vi "MeasConfigType_to_Byte.vi"(4 "MeasConfigType":T1) -> (1 "Byte Array":u8[](array[numeric]))   [LabVIEW 2020, in "Avantes.lvclass"]
uses:
  <instrlib>/Classes/CCD/Avantes/Avantes.lvclass
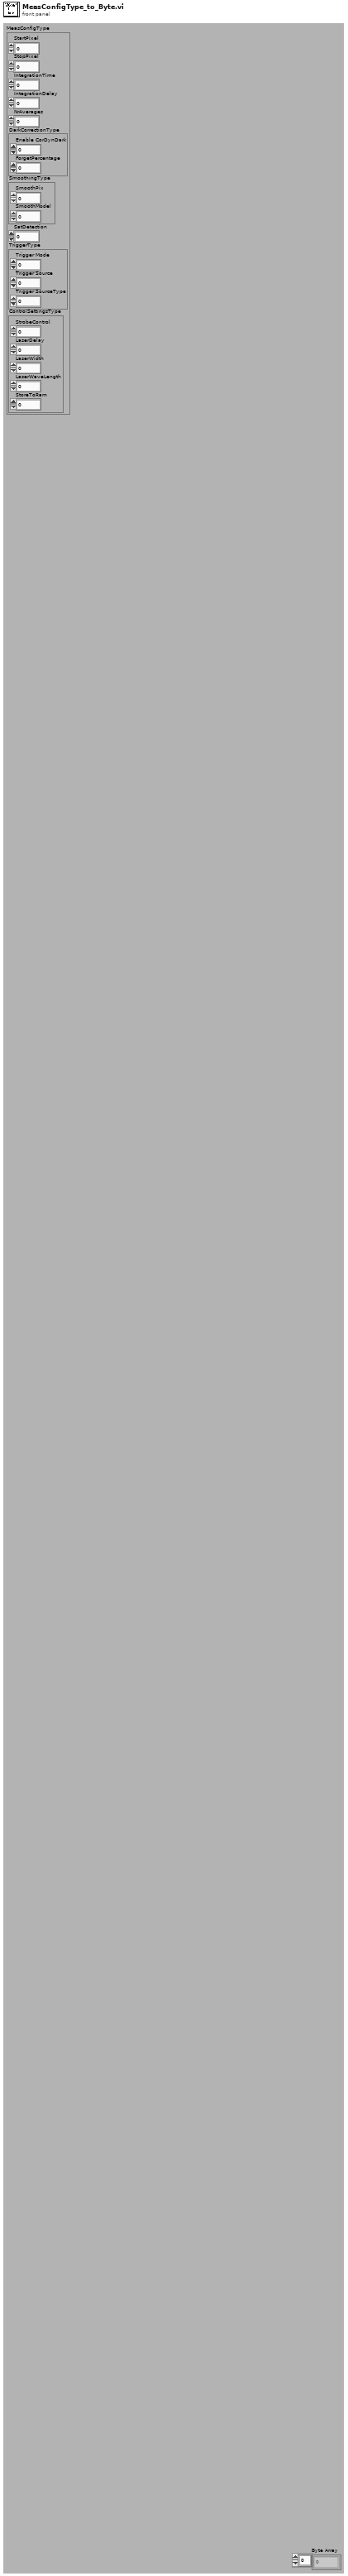
[diagram p1: front panel]
types:
  T1 = cluster{"StartPixel":u16, "StopPixel":u16, "IntegrationTime":sgl, "IntegrationDelay":u32, "NrAverages":u32, "DarkCorrectionType":cluster{"Enable CorDynDark":u8, "ForgetPercentage":u8}, "SmoothingType":cluster{"SmoothPix":u16, "SmoothModel":u8}, "SatDetection":u8, "TriggerType":cluster{"Trigger Mode":u8, "Trigger Source":u8, "Trigger SourceType":u8}, "ControlSettingsType":cluster{"StrobeControl":u16, "LaserDelay":u32, "LaserWidth":u32, "LaserWaveLength":sgl, "StoreToRam":u16}}
  T2 = cluster{"Enable CorDynDark":u8, "ForgetPercentage":u8}
  T3 = cluster{"Trigger Mode":u8, "Trigger Source":u8, "Trigger SourceType":u8}
  T4 = cluster{"StrobeControl":u16, "LaserDelay":u32, "LaserWidth":u32, "LaserWaveLength":sgl, "StoreToRam":u16}
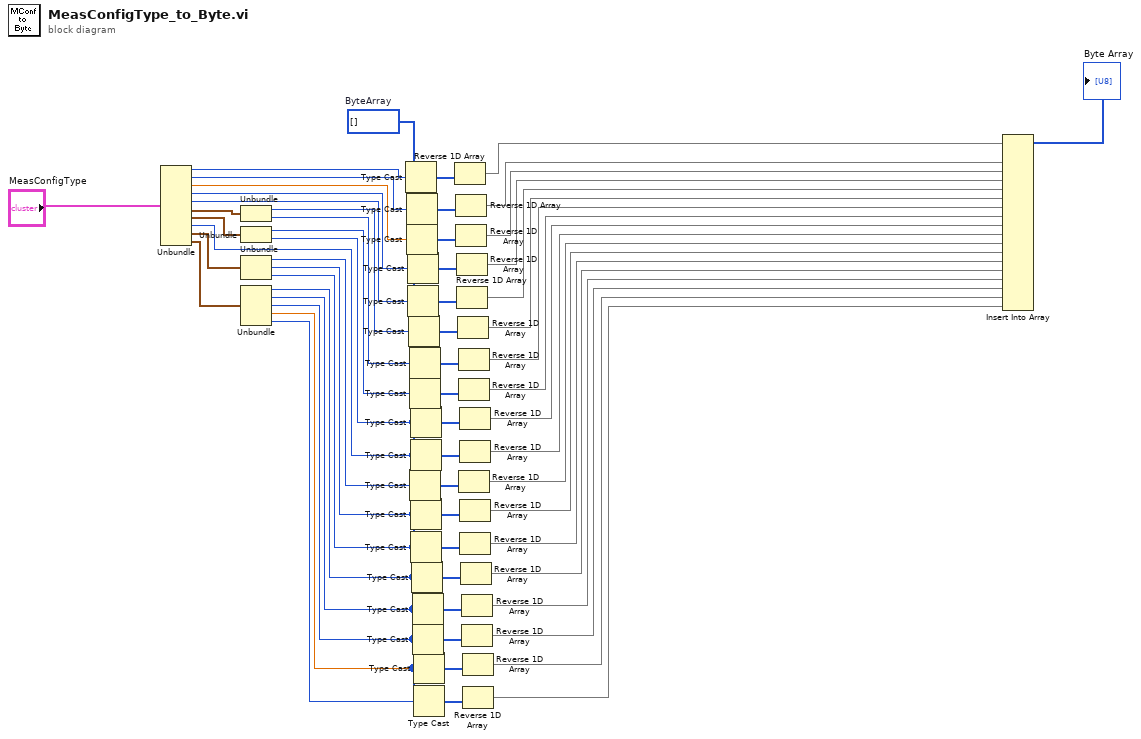
[diagram p0: block diagram]
diagram:
  w3 = u8[] []  # ByteArray
  n1 = Unbundle("MeasConfigType") -> ("StartPixel"=w52:u16, "StopPixel"=w51:u16, "IntegrationTime"=w50:sgl, "IntegrationDelay"=w49:u32, "NrAverages"=w48:u32, "DarkCorrectionType"=w61:T2, "SmoothingType"=w60:cluster{"SmoothPix":u16, "SmoothModel":u8}, "SatDetection"=w38:u8, "TriggerType"=w59:T3, "ControlSettingsType"=w58:T4)
  n2 = Unbundle(w61) -> ("Enable CorDynDark"=w42:u8, "ForgetPercentage"=w41:u8)
  n3 = Unbundle(w60) -> ("SmoothPix"=w40:u16, "SmoothModel"=w39:u8)
  n4 = Unbundle(w59) -> ("Trigger Mode"=w20:u8, "Trigger Source"=w19:u8, "Trigger SourceType"=w18:u8)
  n5 = Unbundle(w58) -> ("StrobeControl"=w17:u16, "LaserDelay"=w16:u32, "LaserWidth"=w15:u32, "LaserWaveLength"=w14:sgl, "StoreToRam"=w13:u16)
  n6 = Type Cast(type=w3, x=w52) -> (*(type *) &x=w53:u8[])
  n7 = Type Cast(type=w3, x=w51) -> (*(type *) &x=w54:u8[])
  n8 = Type Cast(type=w3, x=w50) -> (*(type *) &x=w55:u8[])
  n9 = Type Cast(type=w3, x=w49) -> (*(type *) &x=w56:u8[])
  n10 = Type Cast(type=w3, x=w48) -> (*(type *) &x=w57:u8[])
  n11 = Type Cast(type=w3, x=w42) -> (*(type *) &x=w47:u8[])
  n12 = Type Cast(type=w3, x=w41) -> (*(type *) &x=w46:u8[])
  n13 = Type Cast(type=w3, x=w40) -> (*(type *) &x=w45:u8[])
  n14 = Type Cast(type=w3, x=w20) -> (*(type *) &x=w23:u8[])
  n15 = Type Cast(type=w3, x=w39) -> (*(type *) &x=w44:u8[])
  n16 = Type Cast(type=w3, x=w38) -> (*(type *) &x=w43:u8[])
  n17 = Type Cast(type=w3, x=w19) -> (*(type *) &x=w22:u8[])
  n18 = Type Cast(type=w3, x=w18) -> (*(type *) &x=w21:u8[])
  n19 = Type Cast(type=w3, x=w17) -> (*(type *) &x=w24:u8[])
  n20 = Type Cast(type=w3, x=w16) -> (*(type *) &x=w25:u8[])
  n21 = Type Cast(type=w3, x=w15) -> (*(type *) &x=w26:u8[])
  n22 = Type Cast(type=w3, x=w14) -> (*(type *) &x=w27:u8[])
  n23 = Type Cast(type=w3, x=w13) -> (*(type *) &x=w28:u8[])
  n24 = Reverse 1D Array(array=w53) -> (reversed array=w1:u8[])
  n25 = Reverse 1D Array(array=w54) -> (reversed array=w37:u8[])
  n26 = Reverse 1D Array(array=w55) -> (reversed array=w36:u8[])
  n27 = Reverse 1D Array(array=w56) -> (reversed array=w35:u8[])
  n28 = Reverse 1D Array(array=w57) -> (reversed array=w34:u8[])
  n29 = Reverse 1D Array(array=w47) -> (reversed array=w33:u8[])
  n30 = Reverse 1D Array(array=w46) -> (reversed array=w32:u8[])
  n31 = Reverse 1D Array(array=w45) -> (reversed array=w31:u8[])
  n32 = Reverse 1D Array(array=w23) -> (reversed array=w12:u8[])
  n33 = Reverse 1D Array(array=w44) -> (reversed array=w30:u8[])
  n34 = Reverse 1D Array(array=w43) -> (reversed array=w29:u8[])
  n35 = Reverse 1D Array(array=w22) -> (reversed array=w11:u8[])
  n36 = Reverse 1D Array(array=w21) -> (reversed array=w10:u8[])
  n37 = Reverse 1D Array(array=w24) -> (reversed array=w9:u8[])
  n38 = Reverse 1D Array(array=w25) -> (reversed array=w8:u8[])
  n39 = Reverse 1D Array(array=w26) -> (reversed array=w7:u8[])
  n40 = Reverse 1D Array(array=w27) -> (reversed array=w6:u8[])
  n41 = Reverse 1D Array(array=w28) -> (reversed array=w5:u8[])
  n42 = Insert Into Array(array=w1, new element #1=w37, new element #2=w36, new element #3=w35, new element #4=w34, new element #5=w33, new element #6=w32, new element #7=w31, new element #8=w30, new element #9=w29, new element #10=w12, new element #11=w11, new element #12=w10, new element #13=w9, new element #14=w8, new element #15=w7, new element #16=w6, new element #17=w5) -> (→"Byte Array":u8[])  [unwired: 1 in]
